vi "5492_AutoSpit.vi"(11 "Setting":string="DoYouEvenLift") -> ()   [LabVIEW 2017]
uses:
  5492_LiftButtons.vi
  5492_SpitButton.vi
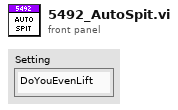
[diagram p1: front panel]
types:
  T1 = typedef "WPI_MotorControlDeviceRef.ctl" = cluster{"DeviceStatus":errorcluster, "Type":T2, "PWM":cluster{"PWM Channel":T3, "DeadBand":T4}, "CAN":cluster{"Device Number":u8, "SetOutput VI Ref":variant, "GetOutput VI Ref":variant, "Enable VI Ref":variant, "Disable VI Ref":variant, "Data":variant}, "Invert":bool, "DIO PWM":cluster{"PWM \"Enable\" Channel":T3, "DIOChannel":T5, "PWM Rate":dbl}}
  T2 = typedef "WPI_MotorControlType.ctl" = enum16{"PWM", "CAN", "DIO PWM"}
  T3 = typedef "FPGA_DIOPWMChannel.ctl" = enum8{"PWM 0", "PWM 1", "PWM 2", "PWM 3", "PWM 4", "PWM 5", "PWM 6", "PWM 7", "PWM 8", "PWM 9", "PWM MXP 0", "PWM MXP 1", "PWM MXP 2", "PWM MXP 3", "PWM MXP 4", "PWM MXP 5", "PWM MXP 6", "PWM MXP 7", "PWM MXP 8", "PWM MXP 9", "Invalid"}
  T4 = typedef "WPI_PWMDeadband.ctl" = cluster{"Name":string, "maxPositivePwm":i32, "minPositivePwm":i32, "centerPwm":i32, "maxNegativePwm":i32, "minNegativePwm":i32, "angularRange":u16}
  T5 = typedef "FPGA_DIOChannel.ctl" = enum8{"DIO 0", "DIO 1", "DIO 2", "DIO 3", "DIO 4", "DIO 5", "DIO 6", "DIO 7", "DIO 8", "DIO 9", "DIO MXP 0", "DIO MXP 1", "DIO MXP 2", "DIO MXP 3", "DIO MXP 4", "DIO MXP 5", "DIO MXP 6", "DIO MXP 7", "DIO MXP 8", "DIO MXP 9", "DIO MXP 10", "DIO MXP 11", "DIO MXP 12", "DIO MXP 13", "DIO MXP 14", "DIO MXP 15", "SPI Port CS1", "SPI Port CS2", "SPI Port CS3", "SPI Port MISO", "SPI Port MOSI", "Invalid"}
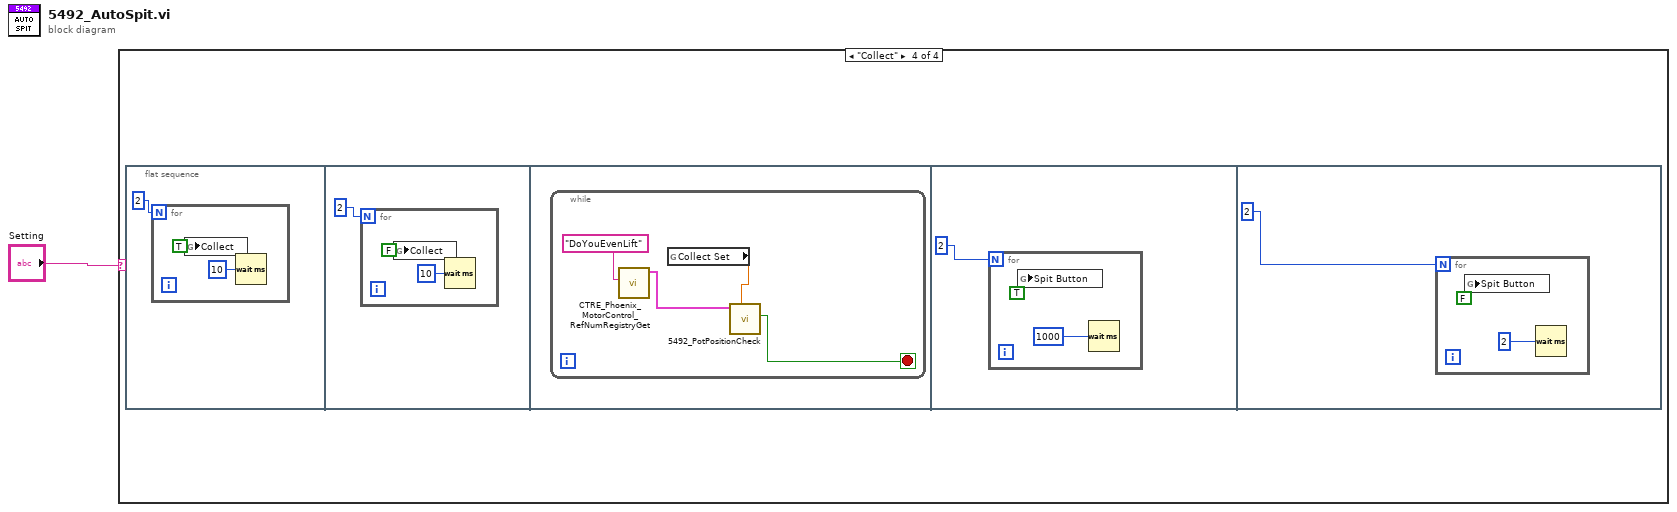
[diagram p0: block diagram]
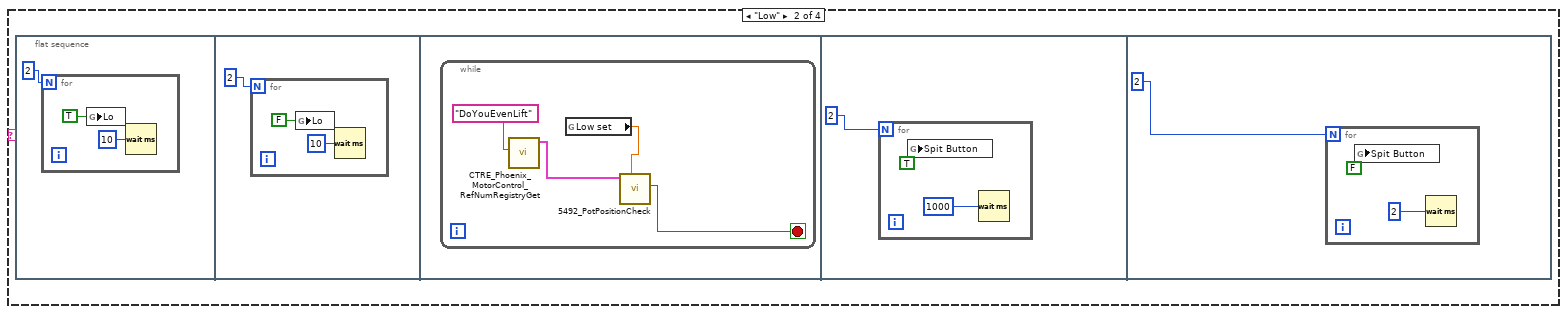
[diagram p3: hidden frame]
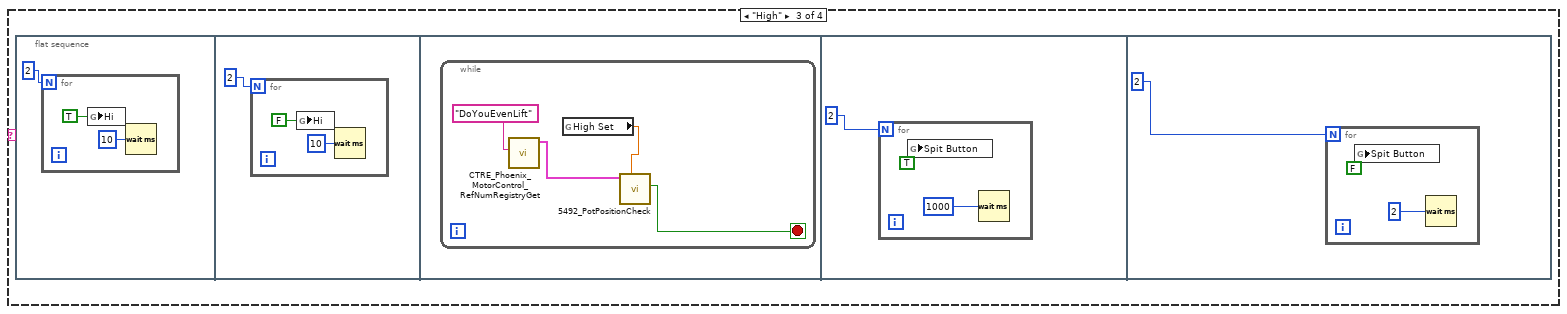
[diagram p4: hidden frame]
diagram:
  n1 = case shown="\"Collect\"" "Setting" {
    frame "False", Default {
    }
    frame "Low" {
      n2 = flat-sequence {
        frame #0 {
          n3 = for {
            N: 2 -> [_]
            n4 = global write "5492_LiftButtons.vi" "Lo"(TRUE ("Lo")) -> ()
            n5 = Wait (ms)(milliseconds to wait=u32 10) -> ()  [unwired: 1 out]
          }
        }
        frame #1 {
          n6 = for {
            N: 2 -> [_]
            n7 = global write "5492_LiftButtons.vi" "Lo"(FALSE ("Lo")) -> ()
            n8 = Wait (ms)(milliseconds to wait=u32 10) -> ()  [unwired: 1 out]
          }
        }
        frame #2 {
          n9 = while {
            stop <- w11 stop-if-true
            n10 = call <vilib>:"CTRE_Phoenix_MotorControl_RefNumRegistryGet.vi"("refnum name"="DoYouEvenLift") -> ("PhoenixMotorControlDevRef"=w10:T1)  [unwired: 9 in, 1 out]
            n11 = global read "5492_LiftButtons.vi" "Low set"() -> (w8:dbl)
            n12 = call "5492_PotPositionCheck.vi"("Position Goal"=w8, "CAN Talon SRX Ref Left"=w10) -> ("Goal Achieved"=w11:bool)  [unwired: 9 in]
          }
        }
        frame #3 {
          n13 = for {
            N: 2 -> [_]
            n14 = global write "5492_SpitButton.vi" "Spit Button"(TRUE ("Lo")) -> ()
            n15 = Wait (ms)(milliseconds to wait=u32 1000) -> ()  [unwired: 1 out]
          }
        }
        frame #4 {
          n16 = for {
            N: 2 -> [_]
            n17 = global write "5492_SpitButton.vi" "Spit Button"(FALSE ("Lo")) -> ()
            n18 = Wait (ms)(milliseconds to wait=u32 2) -> ()  [unwired: 1 out]
          }
        }
      }
    }
    frame "High" {
      n19 = flat-sequence {
        frame #0 {
          n20 = for {
            N: 2 -> [_]
            n21 = global write "5492_LiftButtons.vi" "Hi"(TRUE ("Lo")) -> ()
            n22 = Wait (ms)(milliseconds to wait=u32 10) -> ()  [unwired: 1 out]
          }
        }
        frame #1 {
          n23 = for {
            N: 2 -> [_]
            n24 = global write "5492_LiftButtons.vi" "Hi"(FALSE ("Lo")) -> ()
            n25 = Wait (ms)(milliseconds to wait=u32 10) -> ()  [unwired: 1 out]
          }
        }
        frame #2 {
          n26 = while {
            stop <- w27 stop-if-true
            n27 = call <vilib>:"CTRE_Phoenix_MotorControl_RefNumRegistryGet.vi"("refnum name"="DoYouEvenLift") -> ("PhoenixMotorControlDevRef"=w26:T1)  [unwired: 9 in, 1 out]
            n28 = global read "5492_LiftButtons.vi" "High Set"() -> (w24:dbl)
            n29 = call "5492_PotPositionCheck.vi"("Position Goal"=w24, "CAN Talon SRX Ref Left"=w26) -> ("Goal Achieved"=w27:bool)  [unwired: 9 in]
          }
        }
        frame #3 {
          n30 = for {
            N: 2 -> [_]
            n31 = global write "5492_SpitButton.vi" "Spit Button"(TRUE ("Lo")) -> ()
            n32 = Wait (ms)(milliseconds to wait=u32 1000) -> ()  [unwired: 1 out]
          }
        }
        frame #4 {
          n33 = for {
            N: 2 -> [_]
            n34 = global write "5492_SpitButton.vi" "Spit Button"(FALSE ("Lo")) -> ()
            n35 = Wait (ms)(milliseconds to wait=u32 2) -> ()  [unwired: 1 out]
          }
        }
      }
    }
    frame "Collect" {
      n36 = flat-sequence {
        frame #0 {
          n37 = for {
            N: 2 -> [_]
            n38 = global write "5492_LiftButtons.vi" "Collect"(TRUE ("Lo")) -> ()
            n39 = Wait (ms)(milliseconds to wait=u32 10) -> ()  [unwired: 1 out]
          }
        }
        frame #1 {
          n40 = for {
            N: 2 -> [_]
            n41 = global write "5492_LiftButtons.vi" "Collect"(FALSE ("Lo")) -> ()
            n42 = Wait (ms)(milliseconds to wait=u32 10) -> ()  [unwired: 1 out]
          }
        }
        frame #2 {
          n43 = while {
            stop <- w43 stop-if-true
            n44 = call <vilib>:"CTRE_Phoenix_MotorControl_RefNumRegistryGet.vi"("refnum name"="DoYouEvenLift") -> ("PhoenixMotorControlDevRef"=w42:T1)  [unwired: 9 in, 1 out]
            n45 = global read "5492_LiftButtons.vi" "Collect Set"() -> (w40:dbl)
            n46 = call "5492_PotPositionCheck.vi"("Position Goal"=w40, "CAN Talon SRX Ref Left"=w42) -> ("Goal Achieved"=w43:bool)  [unwired: 9 in]
          }
        }
        frame #3 {
          n47 = for {
            N: 2 -> [_]
            n48 = global write "5492_SpitButton.vi" "Spit Button"(TRUE ("Lo")) -> ()
            n49 = Wait (ms)(milliseconds to wait=u32 1000) -> ()  [unwired: 1 out]
          }
        }
        frame #4 {
          n50 = for {
            N: 2 -> [_]
            n51 = global write "5492_SpitButton.vi" "Spit Button"(FALSE ("Lo")) -> ()
            n52 = Wait (ms)(milliseconds to wait=u32 2) -> ()  [unwired: 1 out]
          }
        }
      }
    }
  }
